vi "counter.vi"() -> ()   [LabVIEW 2020]
panel:
  in  "Reset when more than 50":bool
  in  "Stop Auto Reset Counter":bool
  out "Auto Reset Counter":dbl
  in  "Reset Button":bool
  out "Counter":dbl
  in  "Stop":bool
  # "Counter Auto Reset"
  # "Counter Manual Reset"
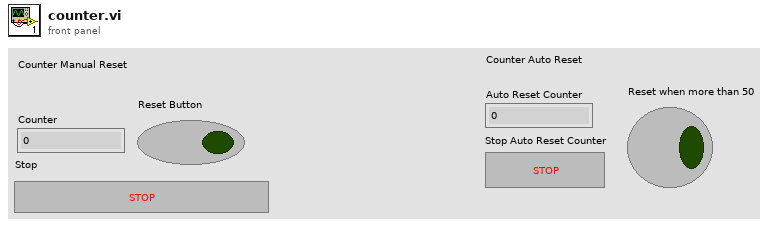
[diagram p1: front panel]
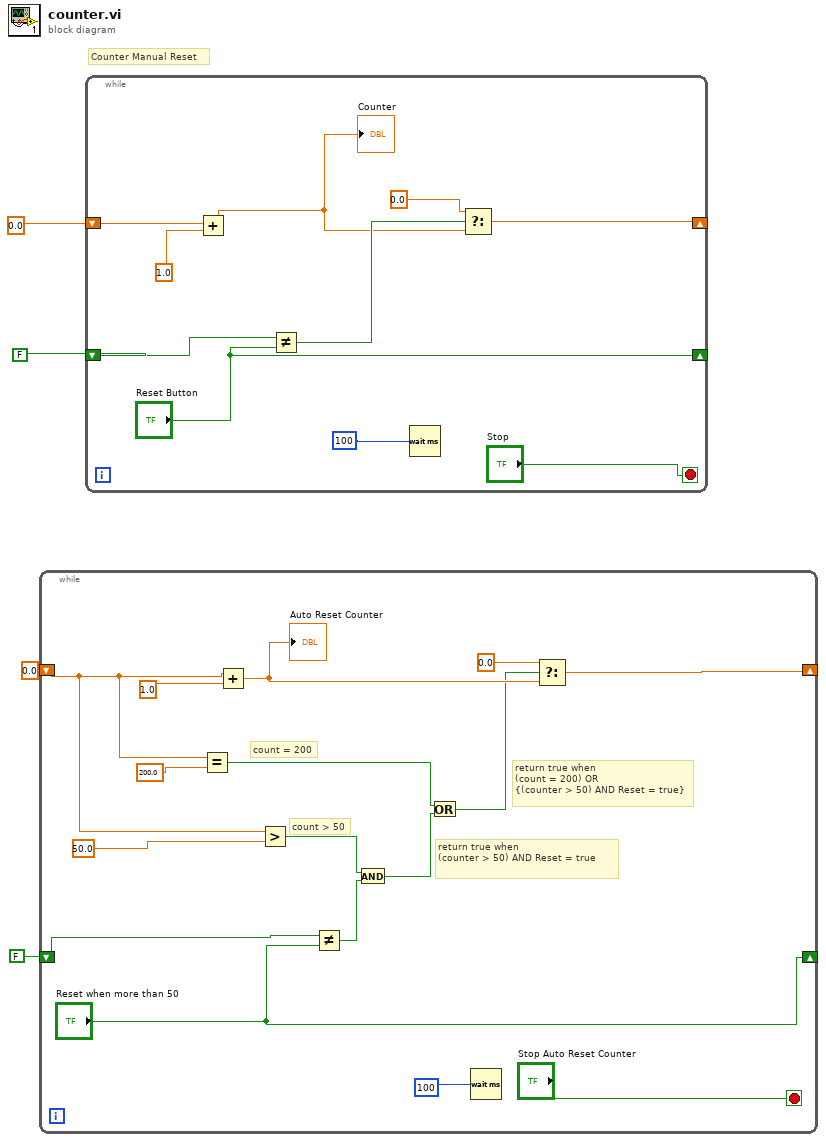
[diagram p0: block diagram]
diagram:
  # "Counter Manual Reset"
  n1 = while {
    shift-right: [w17] -> _
    shift-left: 0.0 -> [w12]
    shift-right: ["Reset when more than 50"] -> _
    shift-left: FALSE -> [w10]
    stop <- "Stop Auto Reset Counter" stop-if-true
    # "return true when\n(count = 200) OR\n{(counter > 50) AND Reset = true}"
    # "return true when \n(counter > 50) AND Reset = true"
    # "count > 50"
    # "count = 200"
    n2 = Equal?(x=w12, y=200.0) -> (x = y?=w7:bool)
    n3 = Add(x=w12, y=1.0) -> (x+y=w15:dbl)
    "Auto Reset Counter" <- w15
    n4 = Greater?(x=w12, y=50.0) -> (0:w9:bool)
    n5 = Not Equal?(x=w10, y="Reset when more than 50") -> (x != y?=w8:bool)
    n6 = And(x=w9, y=w8) -> (x .and. y?=w6:bool)
    n7 = Or(x=w7, y=w6) -> (x .or. y?=w5:bool)
    n8 = Wait (ms)(milliseconds to wait=100) -> ()  [unwired: 1 out]
    n9 = Select(t=0.0, s=w5, f=w15) -> (s? t:f=w17:dbl)
  }
  n10 = while {
    shift-right: [w23] -> _
    shift-left: 0.0 -> [w29]
    shift-right: ["Reset Button"] -> _
    shift-left: FALSE -> [w27]
    stop <- "Stop" stop-if-true
    n11 = Add(x=w29, y=1.0) -> (x+y=w24:dbl)
    "Counter" <- w24
    n12 = Not Equal?(x=w27, y="Reset Button") -> (x != y?=w25:bool)
    n13 = Wait (ms)(milliseconds to wait=100) -> ()  [unwired: 1 out]
    n14 = Select(t=0.0, s=w25, f=w24) -> (s? t:f=w23:dbl)
  }
